vi "Hybrid Main Instrumentation.vi"() -> ()   [LabVIEW 2020]
uses:
  <vilib>/Utility/TDMS File Viewer/NI_TDMS File Viewer.lvlib
panel:
  out "Ignitor Current":dbl(knob) scale=0.0..10.0
  out "Stream Parameters":T1 {"Device Backlog [%]" format="%.2f"}
  out "Actual Scan Rate (Hz)":dbl=1000.0 format="%.3f"
  in  "AIN Range":u8(ring) items=["LJ_rgBIP10V", "LJ_rgBIP1V", "LJ_rgBIPP1V", "LJ_rgBIPP01V"]
  in  "Display Rate (Hz)":i32=1
  in  "Binary":bool
  in  "StreamSettlingFactor":i32
  in  "Resolution Index":u8
  in  "PC buffer size (seconds)":dbl=10.0 format="%.2f"
  in  "Scan Rate (Hz)":dbl=1000.0 format="%.3f"
  out "Oxidizer Mass Flow":dbl(graph)
  out "N2O Tank Mass":dbl(slide) scale=17.0..21.0
  out "Grain Center":dbl(slide) scale=-70.0..40.0
  out "Post-Combustion":dbl(slide) scale=-70.0..40.0
  out "Pre-Combustion":dbl(slide) scale=-70.0..40.0
  out "Injector":dbl(slide) scale=-70.0..40.0
  out "Pressure Chart":dynamicdata(graph)
  out "Thrust Chart":dynamicdata(graph)
  out "Run Tank Pressure":dbl(knob) scale=0.0..10.0
  out "N Flow Pressure":dbl(knob) scale=0.0..10.0
  out "N2O Flow Pressure":dbl(knob) scale=0.0..10.0
  in  "Injector":string
  in  "Orifice Size":string
  in  "File Name":string
  out "Boolean":bool
  in  "START":bool
  in  "[ESC]":bool
  out "Error Message":string
  out "error out":errorcluster
  in  "Folder Path":path
  # "LJ_rgBIP10V\nLJ_rgBIP1V\nLJ_rgBIPP1V\nLJ_rgBIPP01V"
  # "UVR Instrumentation Testing"
  # "Acquires multiple analog input channels over USB from the first found U6."
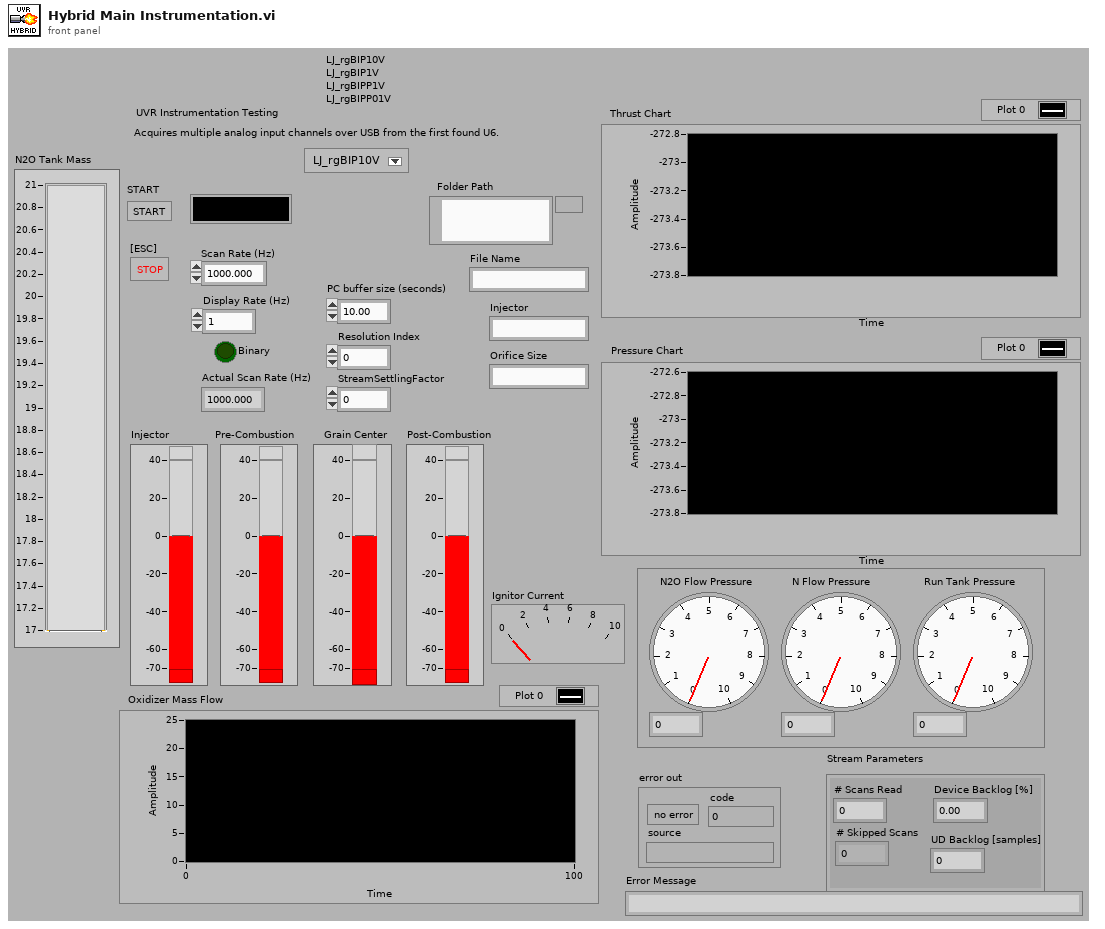
[diagram p1: front panel]
types:
  T1 = cluster{"# Scans Read":i32, "# Skipped Scans":i32, "Device Backlog [%]":dbl, "UD Backlog [samples]":i32}
  T2 = enum16{"open", "open or create", "create or replace", "create", "open (read-only)"}
  T3 = cluster{"PC buffer size (seconds)":dbl, "Resolution Index":u8, "StreamSettlingFactor":i32, "Binary":bool}
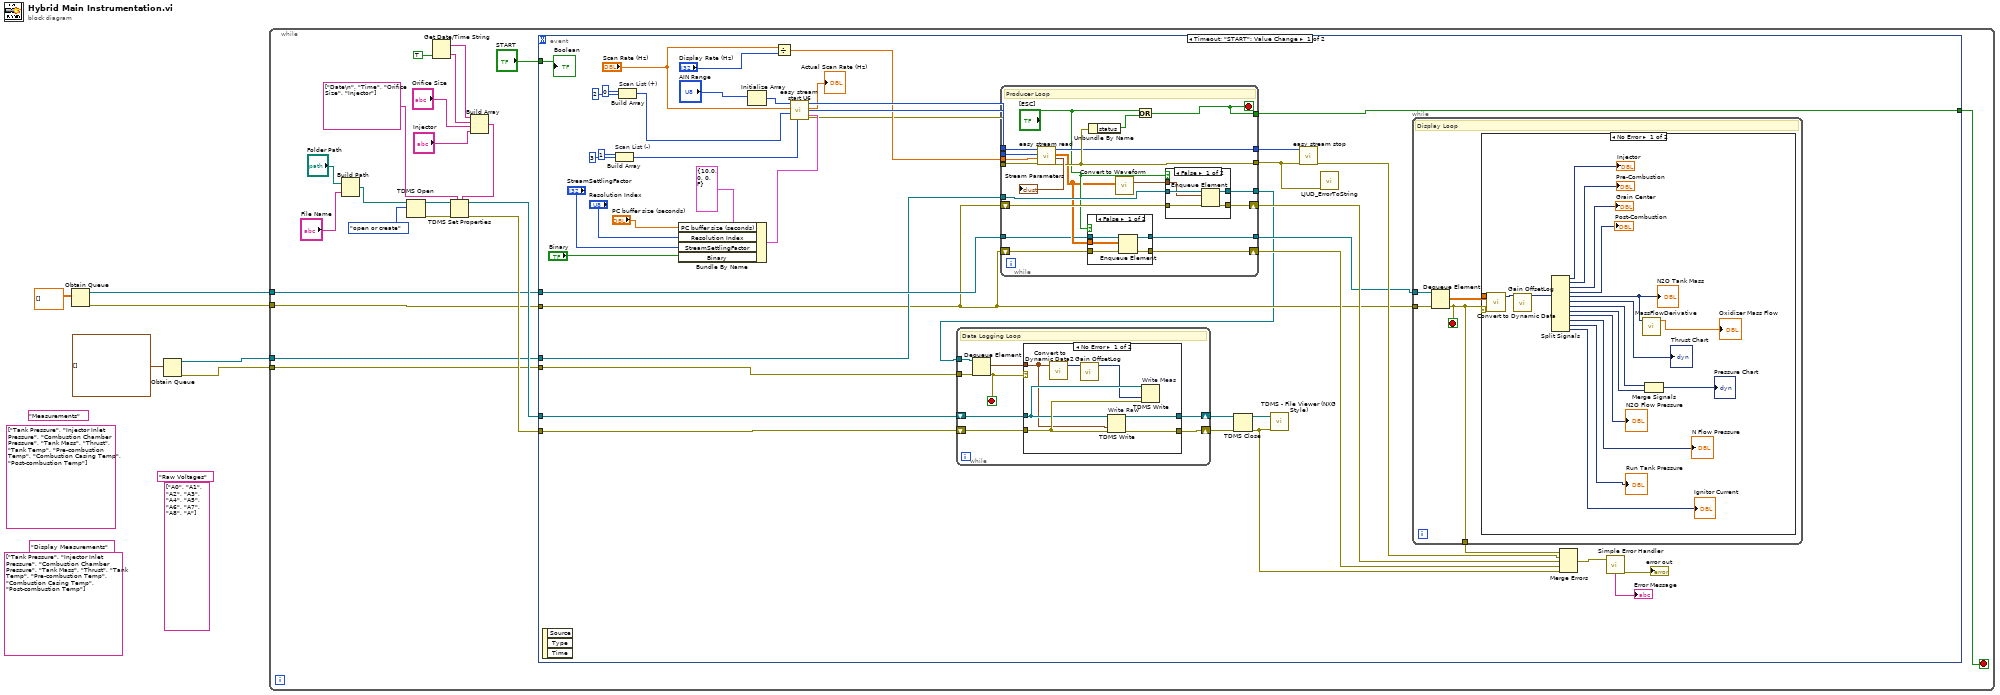
[diagram p0: block diagram]
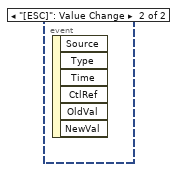
[diagram p6: hidden frame]
diagram:
  (unwired) string[] ["Tank Pressure", "Injector Inlet Pressure", "Combustion Chamber Pressure", "Tank Mass", "Thrust", "Tank Temp", "Pre-combustion Temp", "Combustion Casing Temp", "Post-combustion Temp"] ("property names")
  (unwired) "Display Measurements"
  (unwired) string[] ["Tank Pressure", "Injector Inlet Pressure", "Combustion Chamber Pressure", "Tank Mass", "Thrust", "Tank Temp", "Pre-combustion Temp", "Combustion Casing Temp", "Post-combustion Temp"] ("property names")
  (unwired) "Measurements"
  (unwired) string[] ["A0", "A1", "A2", "A3", "A4", "A5", "A6", "A7", "A8", "A"] ("property names")
  (unwired) "Raw Voltages"
  n1 = Obtain Queue(element data type=dbl[][] []) -> (queue out=w4:refnum<queue>, error out=w3:errorcluster)  [unwired: 4 in, 1 out]
  n2 = Obtain Queue(element data type=waveform(dbl)[] [] ("Waveform")) -> (queue out=w2:refnum<queue>, error out=w1:errorcluster)  [unwired: 4 in, 1 out]
  n3 = while {
    tunnel: w4 -> [w10]
    tunnel: w3 -> [w9]
    tunnel: w2 -> [w8]
    tunnel: w1 -> [w7]
    stop <- w17 stop-if-true
    n4 = Build Path(base path="Folder Path", name or relative path="File Name") -> (appended path=w15:path)
    n5 = TDMS Open(10:T2."open or create" ("operation (0:open)"), 11:w15) -> (0:w27:errorcluster, 3:w26:refnum<k34>)  [unwired: 5 in]
    n6 = Get Date/Time String(want seconds? (F)=TRUE) -> (date string=w24:string, time string=w13:string)  [unwired: 2 in]
    n7 = Build Array(w24, w13, "Orifice Size", "Injector") -> (w22:string[])
    n8 = TDMS Set Properties(5:w22, 7:string[] ["Date\n", "Time", "Orifice Size", "Injector"] ("property names"), 8:w27, 11:w26) -> (0:w19:errorcluster, 3:w20:refnum<k34>)  [unwired: 2 in, 2 out]
    n9 = event shown="[0] Timeout;  \"START\": Value Change" {
      selector: _ -> [_ _]
      dyn-events: _ -> [_ _]
      timeout: _ -> [_ _]
      tunnel: w20 -> [w62 _]
      tunnel: w19 -> [w70 _]
      tunnel: "START" -> [w71 _]
      tunnel: [w68 _] -> w17
      tunnel: w10 -> [w32 _]
      tunnel: w9 -> [w30 _]
      tunnel: w8 -> [w31 _]
      tunnel: w7 -> [w34 _]
      event Timeout; "START": Value Change {
        n10 = event-data() -> ()  [unwired: 1 in, 3 out]
        n11 = Build Array "Scan List (-)"(1 ("SettlingFactor"), 3 ("SettlingFactor")) -> (w47:i32[])
        n12 = Build Array "Scan List (+)"(0 ("SettlingFactor"), 2 ("SettlingFactor")) -> (w50:i32[])
        n13 = Bundle By Name(cluster=T3 {"PC buffer size (seconds)"=10.0, "Resolution Index"=0, "StreamSettlingFactor"=0, "Binary"=FALSE} ("Advanced"), "PC buffer size (seconds)"="PC buffer size (seconds)", "Resolution Index"="Resolution Index", "StreamSettlingFactor"="StreamSettlingFactor", "Binary"="Binary") -> (w56:T3)
        n14 = Initialize Array("AIN Range") -> (w52:u8[])  [unwired: 1 in]
        n15 = Divide(x="Scan Rate (Hz)", y="Display Rate (Hz)") -> (x/y=w41:dbl)
        n16 = call "easy stream start U6.vi"("Advanced"=w56, "Scan List (-)"=w47, "Scan List (+)"=w50, "Scan Rate (Hz)"="Scan Rate (Hz)", "Range Constants"=w52) -> ("error out"=w40:errorcluster, "# Channels"=w42:i32, "Actual Scan Rate (Hz)"=→"Actual Scan Rate (Hz)":dbl, "Handle Out"=w44:i32)  [unwired: 3 in]
        n17 = while {
          tunnel: [w91] -> w68
          shift-right: [w75] -> w66
          shift-left: w30 -> [w90]
          tunnel: w44 -> [w88]
          tunnel: w42 -> [w87]
          tunnel: w41 -> [w86]
          tunnel: w40 -> [w85]
          tunnel: [w82] -> w36
          tunnel: [w80] -> w39
          shift-right: [w74] -> w33
          shift-left: w30 -> [w76]
          tunnel: w31 -> [w89]
          tunnel: w32 -> [w77]
          tunnel: [w73] -> w29
          tunnel: [w72] -> w28
          stop <- w91 stop-if-true
          # "Producer Loop"
          n18 = call "easy stream read.vi"("error in"=w85, "Scans To Read"=w86, "# Channels In Stream"=w87, "Handle In"=w88) -> ("error out"=w82:errorcluster, "Stream Parameters"=→"Stream Parameters":T1, "Data"=w78:dbl[][], "Handle Out"=w80:i32)  [unwired: 4 in]
          n19 = case shown="False" "[ESC]" {
            tunnel: w78 -> [w96 _]
            tunnel: w77 -> [w95 w98]
            tunnel: w76 -> [w94 w97]
            tunnel: [w93 w97] -> w74
            tunnel: [w92 w98] -> w73
            frame False {
              n20 = Enqueue Element(queue=w95, element=w96, error in (no error)=w94) -> (queue out=w92:refnum<queue>, error out=w93:errorcluster)  [unwired: 1 in, 1 out]
            }
            frame True {
            }
          }
          n21 = Unbundle By Name(w82) -> ("status"=w81:bool)
          n22 = call "Convert to Waveform.vi"("Data"=w78) -> ("Waveform"=w83:waveform(dbl)[])  [unwired: 10 in]
          n23 = Or(x="[ESC]", y=w81) -> (x .or. y?=w91:bool)
          n24 = case shown="False" "[ESC]" {
            tunnel: w89 -> [w103 w105]
            tunnel: [w99 w105] -> w72
            tunnel: [w102 w104] -> w75
            tunnel: w90 -> [w101 w104]
            tunnel: w83 -> [w100 _]
            frame False {
              n25 = Enqueue Element(queue=w103, element=w100, error in (no error)=w101) -> (queue out=w99:refnum<queue>, error out=w102:errorcluster)  [unwired: 1 in, 1 out]
            }
            frame True {
            }
          }
        }
        n26 = while {
          shift-right: [w112] -> w64
          shift-left: w62 -> [w109]
          shift-right: [w111] -> w63
          shift-left: w70 -> [w113]
          tunnel: w28 -> [w107]
          tunnel: w34 -> [w106]
          stop <- w110 stop-if-true
          # "Data Logging Loop"
          n27 = Dequeue Element(queue=w107, error in (no error)=w106) -> (element=w108:waveform(dbl)[], error out=w110:errorcluster)  [unwired: 1 in, 2 out]
          n28 = case shown="No Error" w110 {
            tunnel: w109 -> [w117 w122]
            tunnel: w113 -> [w119 w121]
            tunnel: [w120 w122] -> w112
            tunnel: [w118 w121] -> w111
            tunnel: w108 -> [w114 _]
            frame No Error {
              n29 = call "Convert to Dynamic Data2"("Array of Waveforms"=w114) -> ("Dynamic Data Type"=w115:dynamicdata)  [unwired: 3 in]
              n30 = call "Gain OffsetLog.vi"("Dynamic Data"=w115) -> ("Dynamic Data"=w116:dynamicdata)  [unwired: 14 in]
              n31 = TDMS Write "Write Raw"(0:w117, 9:w114, 11:w119) -> (4:w120:refnum<k34>, 15:w118:errorcluster)  [unwired: 3 in, 2 out]
              n32 = TDMS Write "Write Meas"(0:w117, 9:w116, 11:w119) -> ()  [unwired: 3 in, 4 out]
            }
            frame Error {
            }
          }
        }
        n33 = TDMS Close(8:w63, 11:w64) -> (0:w35:errorcluster, 3:w37:path)
        n34 = call <vilib>:"TDMS - File Viewer (NXG Style).vi"("error in"=w35, "file in"=w37) -> ()  [unwired: 8 in, 2 out]
        n35 = call "easy stream stop.vi"("error in"=w36, "Handle In"=w39) -> ("error out"=w38:errorcluster)  [unwired: 7 in, 2 out]
        n36 = call "LJUD_ErrorToString.vi"("error in"=w36) -> ()  [unwired: 10 in, 1 out]
        n37 = while "Display Loop" {
          tunnel: [w125] -> w65
          tunnel: w29 -> [w124]
          tunnel: w30 -> [w123]
          stop <- w125 stop-if-true
          # "Display Loop"
          n38 = Dequeue Element(queue=w124, error in (no error)=w123) -> (element=w126:dbl[][], error out=w125:errorcluster)  [unwired: 1 in, 2 out]
          n39 = case shown="No Error" w125 {
            tunnel: w126 -> [w142 _]
            frame No Error {
              n40 = call "Convert to Dynamic Data"("2D Array"=w142) -> ("Dynamic Data Type"=w140:dynamicdata)  [unwired: 3 in]
              n41 = call "Gain OffsetLog.vi"("Dynamic Data"=w140) -> ("Dynamic Data"=w141:dynamicdata)  [unwired: 14 in]
              n42 = Split Signals(w141) -> (→"Injector":dynamicdata, →"Pre-Combustion":dynamicdata, →"Grain Center":dynamicdata, →"Post-Combustion":dynamicdata, w134:dynamicdata, →"Thrust Chart":dynamicdata, w132:dynamicdata, w131:dynamicdata, →"N2O Flow Pressure":dynamicdata, →"N Flow Pressure":dynamicdata, →"Run Tank Pressure":dynamicdata, →"Ignitor Current":dynamicdata)  [unwired: 12 in]
              "N2O Tank Mass" <- w134
              n43 = call "MassFlowDerivative.vi"("Dynamic Data"=w134) -> ("Filtered x"=→"Oxidizer Mass Flow":dbl)  [unwired: 10 in]
              n44 = Merge Signals(w132, w131) -> (→"Pressure Chart":dynamicdata)
            }
            frame Error {
            }
          }
        }
        n45 = Merge Errors(w65, w38, w66, w33, w35) -> (w69:errorcluster)
        n46 = call <vilib>:"Simple Error Handler.vi"("error in (no error)"=w69) -> ("error out"=→"error out":errorcluster, "message"=→"Error Message":string)  [unwired: 4 in, 3 out]
        "Boolean" <- w71
      }
      event "[ESC]": Value Change {
        n47 = event-data() -> ()  [unwired: 1 in, 6 out]
      }
    }
  }
